vi "JKISM++ Request JKISM to Broadcast Status Change.vi"(7 "Module Name":string, 8 "Error In (no error)":errorcluster, 10 "Arguments (\"\")":string, 11 "Status":string="DoA") -> (0 "error out":errorcluster)   [LabVIEW 2014, in "JKI State Machine++.lvlib"]
doc: "Request JKISM to publish status change to JKISM specified. This is usually used in sub-loops with a JKISM for acting as a holistic module.\n\n<b>Inputs:</b>\n - <b>Status</b>: status to broadcast.\n - <b>Arguments (\"\")</b>: Argument of the status.\n - <b>Module Name</b>:Host Module Name\n - <b>Error In (no error)</b>: Error cluster\n\n<b>Outputs:</b>\n - <b>error out</b>: Error cluster"
uses:
  JKI State Machine++.lvlib
  _Support/JKISMQ/_JKISMQFGVOPER.ctl
  _Support/Typedef/_Cross JKISM State Data.ctl
  _Support/Typedef/_JKISM_MSG_TYPE.ctl
  _Support/Typedef/_Cross JKISM State Response.ctl
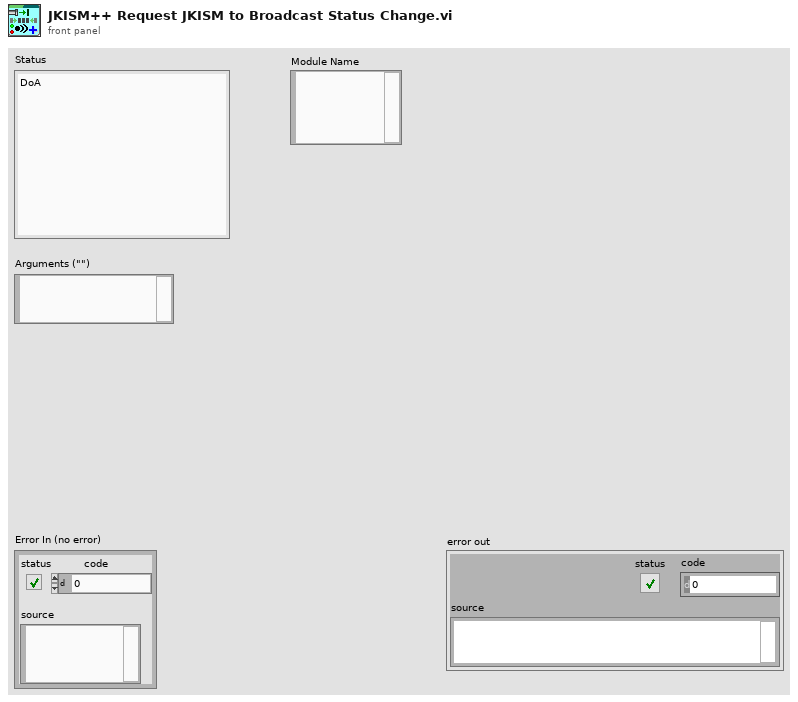
[diagram p1: front panel]
types:
  T1 = typedef "JKI State Machine++.lvlib/_JKISM_MSG_TYPE.ctl" = enum16{"Sync Message(-@)", "Async Message(->)", "Async without Response(->|)", "Async Response", "Broadcast(-><status>)", "Broadcast(-><interrupt>)", "Request to Post Message", "Request to Post Message without Reply", "Request to Publish Status"}
  T2 = typedef "JKI State Machine++.lvlib/_Cross JKISM State Data.ctl" = cluster{"Msg Type":T1, "state":string, "args":string, "source":string, "RespQ":refnum<queue>, "Pre-State":string, "Arg-State":string, "Target":string}
  T3 = typedef "JKI State Machine++.lvlib/_JKISMQFGVOPER.ctl" = enum16{"Get By Name", "List", "Check If Name Exists", "Release", "Module Status"}
  T4 = typedef "JKI State Machine++.lvlib/_JKISMQ.ctl" = cluster{"Module Name":string, "Queue":refnum<queue>, "Locked Status":refnum<data-value>, "Mode":T5, "User Event":refnum<user-event>, "Queue Count":i32}
  T5 = typedef "JKI State Machine++.lvlib/_JKISM_MODE.ctl" = enum16{"Stand Alone", "JKISM", "Action Worker"}
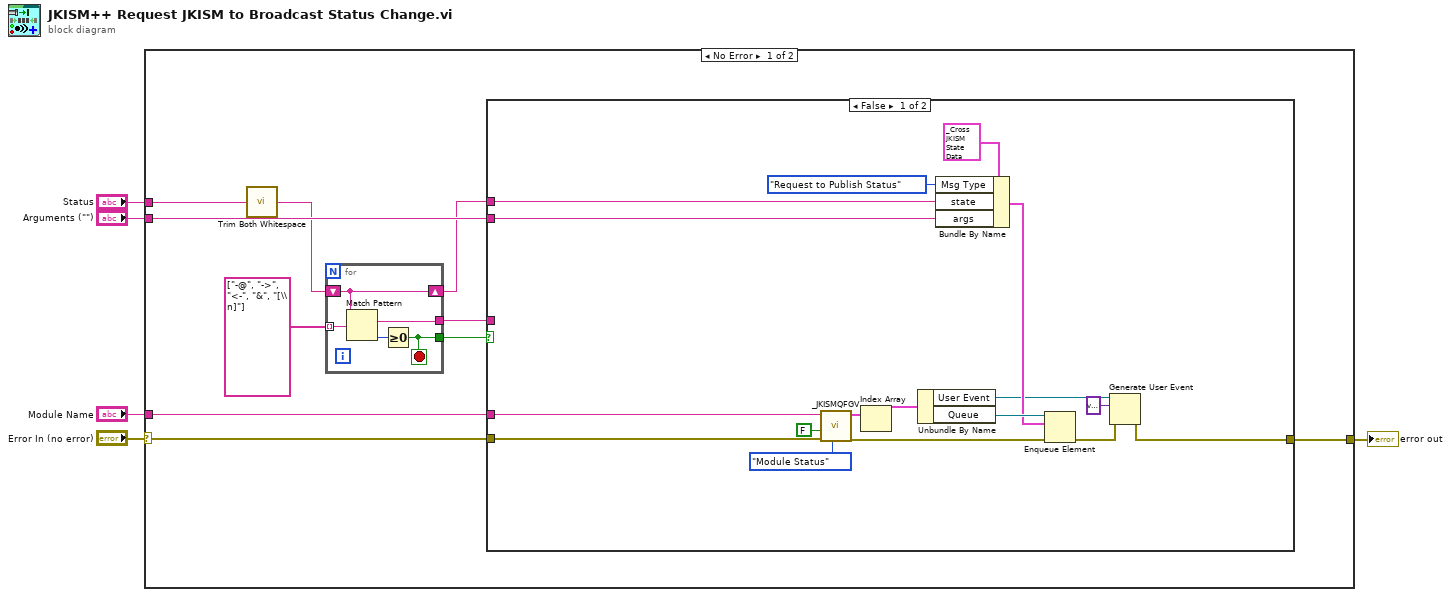
[diagram p0: block diagram]
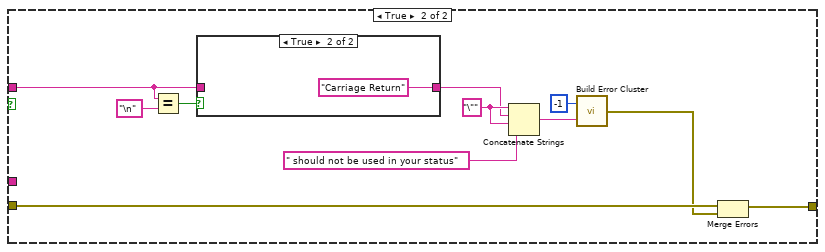
[diagram p2: hidden frame]
diagram:
  n1 = case shown="No Error" "Error In (no error)" {
    selector: "Error In (no error)" -> [w14 w51]
    tunnel: "Status" -> [w12 _]
    tunnel: [w15 w51] -> w3
    tunnel: "Arguments (\"\")" -> [w13 _]
    tunnel: "Module Name" -> [w11 _]
    frame No Error {
      n2 = call "Trim Both Whitespace.vi"("string"=w12) -> ("trimmed string"=w6:string)  [unwired: 1 in]
      n3 = for {
        shift-right: [w50] -> w9
        shift-left: w6 -> [w50]
        tunnel: string[] ["-@", "->", "<-", "&", "[\\n]"] -> [w49] mode=indexing
        tunnel: [w47] -> w7
        tunnel: [w46] -> w8
        stop <- w46 stop-if-true
        n4 = Match Pattern(string=w50, regular expression=w49) -> (match substring=w47:string, offset past match=w48:i32)  [unwired: 1 in, 2 out]
        n5 = Greater Or Equal To 0?(x=w48) -> (x >= 0?=w46:bool)
      }
      n6 = case shown="False" w8 {
        tunnel: w13 -> [w24 _]
        tunnel: [w16 w35] -> w15
        tunnel: w14 -> [w22 w36]
        tunnel: w9 -> [w25 _]
        tunnel: w7 -> [_ w33]
        tunnel: w11 -> [w21 _]
        frame False {
          n7 = call "_JKISMQFGV.vi"("Operation"=_JKISMQFGVOPER."Module Status", "Error in"=w22, "create if not found? (T)"=FALSE, "Name(\"\" to use uuid) in"=w21) -> ("Error out"=w23:errorcluster, "Array"=w31:T4[])  [unwired: 4 in, 2 out]
          n8 = Index Array(array=w31) -> (element=w30:T4)  [unwired: 1 in]
          n9 = Unbundle By Name(w30) -> ("User Event"=w18:refnum<user-event>, "Queue"=w29:refnum<queue>)
          n10 = Bundle By Name(cluster=T2 {"Msg Type"=enum."Sync Message(-@)", "state"="", "args"="", "source"="", "RespQ"=refnum, "Pre-State"="", "Arg-State"="", "Target"=""} ("element"), "Msg Type"=_JKISM_MSG_TYPE."Request to Publish Status", "state"=w25, "args"=w24) -> (w27:T2)
          n11 = Enqueue Element(queue=w29, element=w27, error in (no error)=w23) -> (error out=w17:errorcluster)  [unwired: 1 in, 2 out]
          n12 = Generate User Event(user event=w18, event data cluster=variant ("event data"), error in=w17) -> (error out=w16:errorcluster)  [unwired: 1 in, 1 out]
        }
        frame True {
          w40 = "\"" ("string")
          n13 = Equal?(x=w33, y="\n" ("regular expression")) -> (x = y?=w37:bool)
          n14 = case shown="True" w37 {
            tunnel: [w44 "Carriage Return" ("State")] -> w39
            tunnel: w33 -> [w44 _]
            frame False {
            }
            frame True {
            }
          }
          n15 = Concatenate Strings(w40, w39, w40, " should not be used in your status" ("String to Prepend to source (\"\")")) -> (w41:string)
          n16 = call "Build Error Cluster.vi"("String to Prepend to source (\"\")"=w41, "code"=-1) -> ("error out"=w34:errorcluster)
          n17 = Merge Errors(w36, w34) -> (w35:errorcluster)
        }
      }
    }
    frame Error {
    }
  }
  "error out" <- w3
